vi "GetRaster_bu.vi"(0 "Galvo Array":refnum<class "Galvonometer.lvclass">[](array[class]), 1 "Scan.lvclass":refnum<class "Scan.lvclass">, 5 "error in (no error)":errorcluster) -> (15 "Galvo Array":dbl[][](array[numeric]), 19 "error IO":errorcluster)   [LabVIEW 2017]
uses:
  classes/Scans/Scan.lvclass
  classes/HardwareObjects/Galvonometer/Galvonometer.lvclass
  classes/Scans/Scan.lvclass/Scan.ctl
  classes/HardwareObjects/Galvonometer/Galvonometer.lvclass/Galvonometer.ctl
  classes/Scans/Read A scans.vi
  classes/Scans/Read B scans.vi
  classes/Scans/Read Bidirectional.vi
  classes/Scans/Read C scans.vi
  classes/Scans/Read Repeat B scans.vi
  classes/Scans/Read Scan Angle (degrees).vi
  classes/Scans/Read Scan Pattern.vi
  classes/Scans/Read X FOV (degrees).vi
  classes/Scans/Read X offset (degrees).vi
  classes/Scans/Read Y FOV (degrees).vi
  classes/Scans/Read Y offset (degrees).vi
  <vilib>/Analysis/1siggen.llb/Ramp Pattern by Samples.vi
  classes/HardwareObjects/Galvonometer/Read Output Scale Factor (V_degrees).vi
  <vilib>/Utility/file.llb/Write Delimited Spreadsheet (DBL).vi
  <vilib>/Analysis/NI_AALBase.lvlib
panel:
  in  "Read scan parameters":bool
  in  "Display Raster":bool
  out "Y offset (degrees)":dbl
  out "Y FOV (degrees)":dbl
  out "X offset (degrees)":dbl
  out "X FOV (degrees)":dbl
  out "Scan Pattern":string
  out "Scan Angle (degrees)":dbl
  out "Repeat B scans":dbl
  out "C scans":dbl
  out "Bidirectional":bool
  out "B scans":dbl
  out "A scans":dbl
  out "Raster":dbl[][](graph)
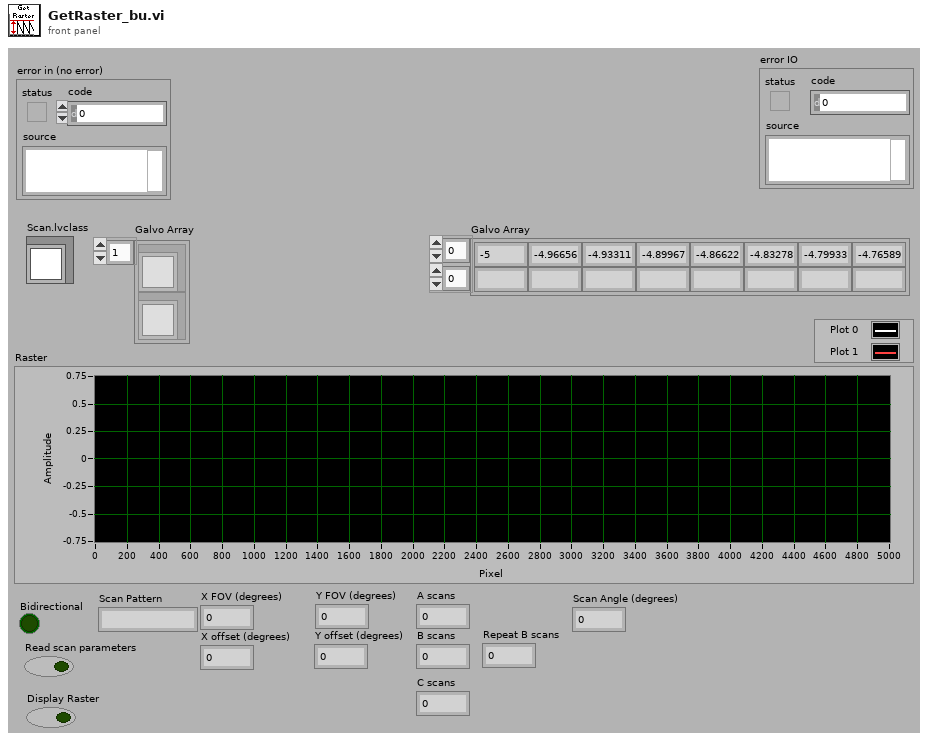
[diagram p1: front panel]
types:
  T1 = cluster{"X FOV (degrees)":dbl, "X offset (degrees)":dbl, "Y FOV (degrees)":dbl, "Y offset (degrees)":dbl}
  T2 = cluster{"X FOV (degrees)":dbl, "Y FOV (degrees)":dbl}
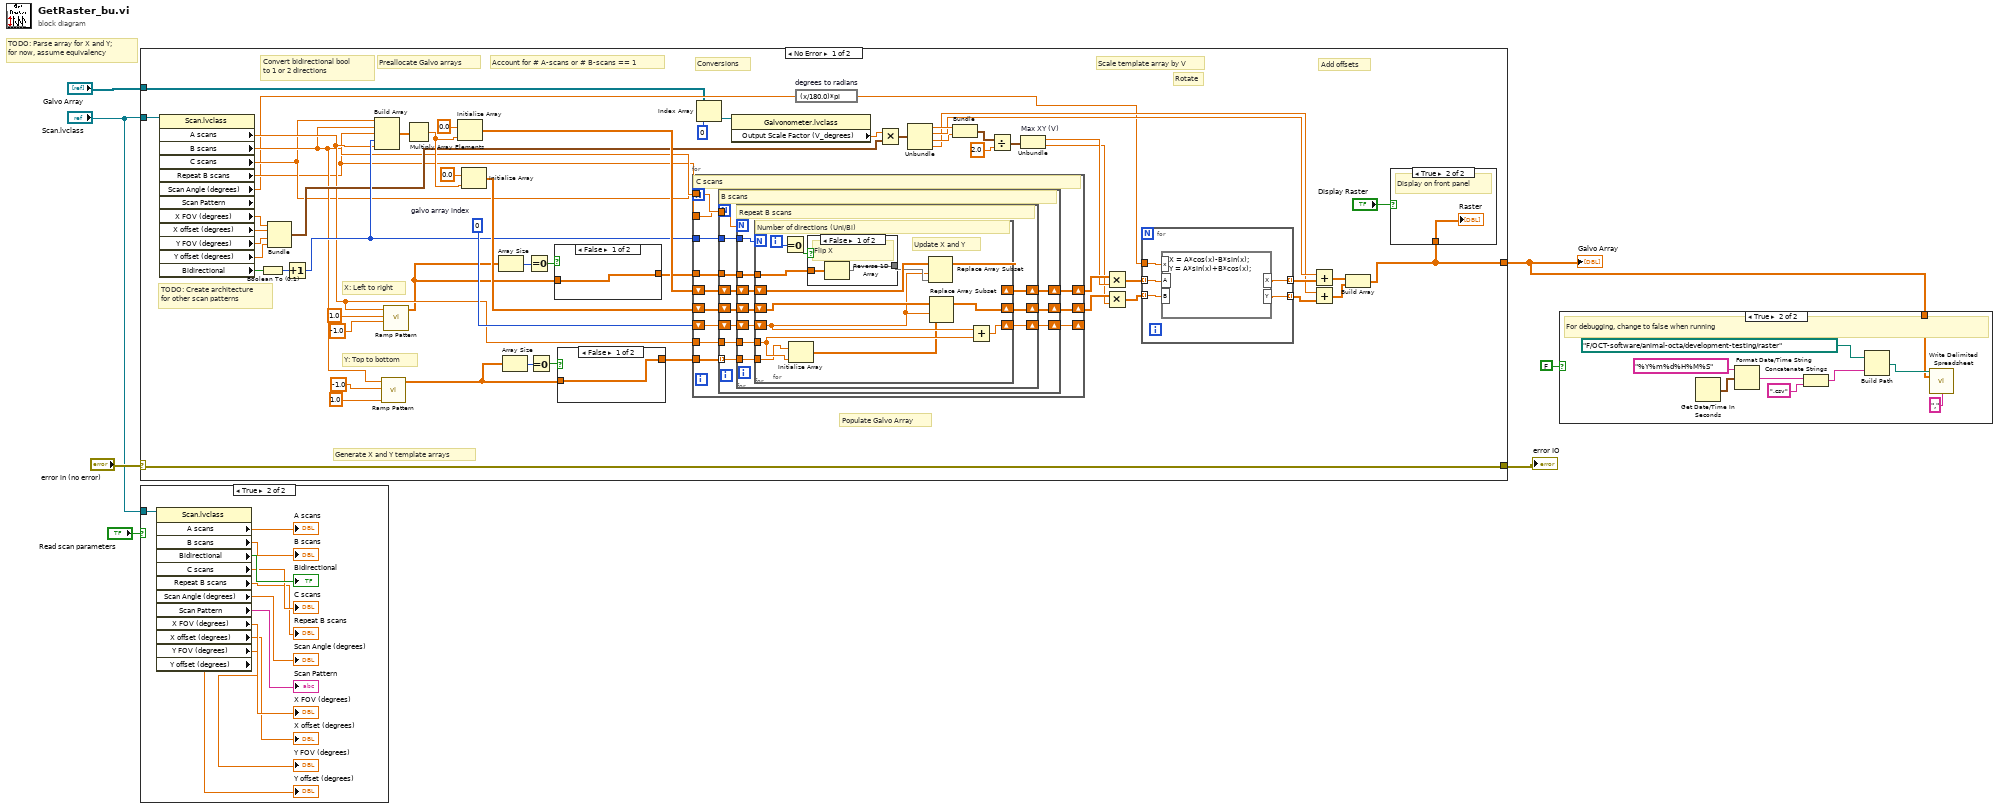
[diagram p0: block diagram]
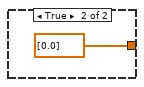
[diagram p3: hidden frame]
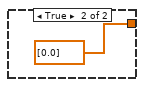
[diagram p4: hidden frame]
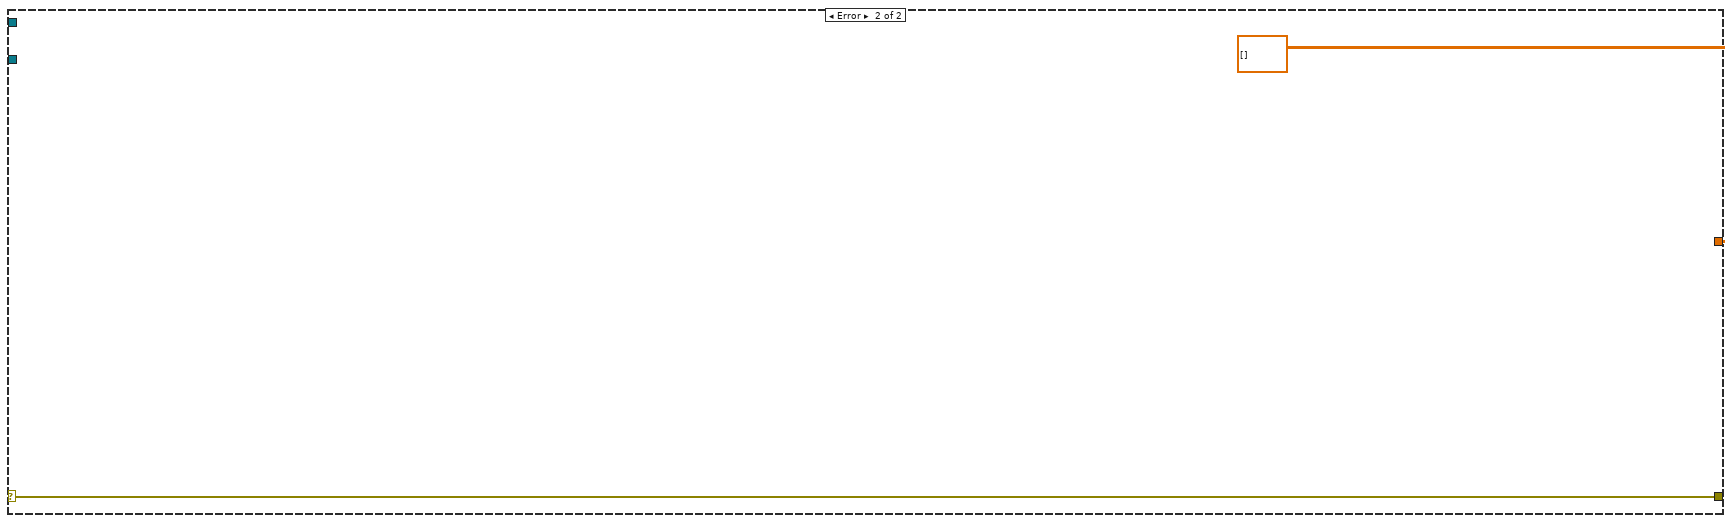
[diagram p7: hidden frame]
diagram:
  # "TODO: Parse array for X and Y;\nfor now, assume equivalency"
  n1 = case shown="No Error" "error in (no error)" {
    selector: "error in (no error)" -> [w66 w127]
    tunnel: [w66 w127] -> w7
    tunnel: [w9 dbl[][] []] -> w2
    tunnel: "Scan.lvclass" -> [w31 _]
    tunnel: "Galvo Array" -> [w22 _]
    frame No Error {
      w58 = 0  # galvo array index
      # "Account for # A-scans or # B-scans == 1"
      # "TODO: Create architecture\nfor other scan patterns"
      # "Convert bidirectional bool\nto 1 or 2 directions"
      # "Conversions"
      # "Add offsets"
      # "Rotate"
      # "Scale template array by V"
      # "Populate Galvo Array"
      # "Preallocate Galvo arrays"
      # "Y: Top to bottom"
      # "X: Left to right"
      # "Generate X and Y template arrays"
      n2 = property class="Scan.lvclass" props=["A scans", "B scans", "C scans", "Repeat B scans", "Scan Angle (degrees)", "Scan Pattern", "X FOV (degrees)", "X offset (degrees)", "Y FOV (degrees)", "Y offset (degrees)", "Bidirectional"](reference=w31) -> ("A scans"=w28:dbl, "B scans"=w27:dbl, "C scans"=w26:dbl, "Repeat B scans"=w25:dbl, "Scan Angle (degrees)"=w24:dbl, "X FOV (degrees)"=w32:dbl, "X offset (degrees)"=w33:dbl, "Y FOV (degrees)"=w34:dbl, "Y offset (degrees)"=w35:dbl, "Bidirectional"=w36:bool)  [unwired: 1 in, 3 out]
      n3 = Boolean To (0,1)(Boolean=w36) -> (0, 1=w37:i16)
      n4 = Bundle("X FOV (degrees)"=w32, "X offset (degrees)"=w33, "Y FOV (degrees)"=w34, "Y offset (degrees)"=w35) -> (w29:T1)  [unwired: 1 in]
      n5 = Increment(x=w37) -> (x+1=w30:i16)
      n6 = Build Array(w26, w27, w25, w30, w28) -> (w60:dbl[])
      n7 = call-poly <vilib>:"Ramp Pattern.vi"("start"=1.0, "end"=-1.0, "samples"=w27) -> ("Ramp Pattern"=w15:dbl[])  [unwired: 7 in, 1 out]
      n8 = call-poly <vilib>:"Ramp Pattern.vi"("start"=-1.0, "end"=1.0, "samples"=w28) -> ("Ramp Pattern"=w10:dbl[])  [unwired: 7 in, 1 out]
      n9 = Multiply Array Elements(1:w60) -> (0:w56:dbl)
      n10 = Initialize Array(0.0 ("element"), w56) -> (w59:dbl[])
      n11 = Initialize Array(0.0 ("element"), w56) -> (w55:dbl[])
      n12 = Array Size(array=w10) -> (size(s)=w12:i32)
      n13 = Array Size(array=w15) -> (size(s)=w16:i32)
      n14 = Equal To 0?(x=w12) -> (x = 0?=w11:bool)
      n15 = Equal To 0?(x=w16) -> (x = 0?=w17:bool)
      n16 = case shown="False" w11 {
        tunnel: w10 -> [w67 _]
        tunnel: [w67 dbl[] [0.0] ("Ramp Pattern")] -> w13
        frame False {
        }
        frame True {
        }
      }
      n17 = case shown="False" w17 {
        tunnel: w15 -> [w69 _]
        tunnel: [w69 dbl[] [0.0] ("Ramp Pattern")] -> w14
        frame False {
        }
        frame True {
        }
      }
      n18 = for {
        N: w26 -> [_]
        tunnel: w27 -> [w88]
        tunnel: w25 -> [w87]
        tunnel: w30 -> [w86]
        tunnel: w13 -> [w84]
        tunnel: w28 -> [w82]
        shift-right: [w78] -> _
        shift-left: w58 -> [w83]
        shift-right: [w81] -> w54
        shift-left: w59 -> [w85]
        shift-right: [w79] -> w53
        shift-left: w55 -> [w80]
        tunnel: w14 -> [w77]
        # "C scans"
        n19 = for {
          N: w88 -> [_]
          tunnel: w87 -> [w99]
          tunnel: w86 -> [w98]
          tunnel: w84 -> [w97]
          tunnel: w82 -> [w95]
          shift-right: [w91] -> w78
          shift-left: w83 -> [w96]
          shift-right: [w94] -> w81
          shift-left: w85 -> [w89]
          shift-right: [w92] -> w79
          shift-left: w80 -> [w93]
          tunnel: w77 -> [w90] mode=indexing
          # "B scans"
          n20 = for {
            N: w99 -> [_]
            tunnel: w98 -> [w109]
            tunnel: w97 -> [w108]
            tunnel: w95 -> [w106]
            shift-right: [w102] -> w91
            shift-left: w96 -> [w107]
            shift-right: [w105] -> w94
            shift-left: w89 -> [w100]
            shift-right: [w103] -> w92
            shift-left: w93 -> [w104]
            tunnel: w90 -> [w101]
            # "Repeat B scans"
            n21 = for {
              N: w109 -> [_]
              tunnel: w108 -> [w120]
              shift-right: [w115] -> w105
              shift-left: w100 -> [w119]
              tunnel: w106 -> [w117]
              shift-right: [w118] -> w102
              shift-left: w107 -> [w112]
              shift-right: [w113] -> w103
              shift-left: w104 -> [w114]
              tunnel: w101 -> [w111]
              i -> [w122]
              # "Update X and Y"
              # "Number of directions (Uni/Bi)"
              n22 = Equal To 0?(x=w122) -> (x = 0?=w121:bool)
              n23 = Initialize Array(w111, w117) -> (w110:dbl[])
              n24 = case shown="False" w121 {
                tunnel: w120 -> [w124 w125]
                tunnel: [w123 w125] -> w116
                frame False {
                  # "Flip X"
                  n25 = Reverse 1D Array(array=w124) -> (reversed array=w123:dbl[])
                }
                frame True {
                  # "Leave X as is"
                }
              }
              n26 = Replace Array Subset(array=w119, new element=w116, index=w112) -> (w115:dbl[])
              n27 = Replace Array Subset(array=w114, new element=w110, index=w112) -> (w113:dbl[])
              n28 = Add(x=w112, y=w117) -> (x+y=w118:dbl)
            }
          }
        }
      }
      n29 = Index Array(array=w22, index=0) -> (element=w23:refnum<class "Galvonometer.lvclass">)
      n30 = property class="Galvonometer.lvclass"(reference=w23) -> ("Output Scale Factor (V_degrees)"=w20:dbl)  [unwired: 1 in, 2 out]
      n31 = expression code="(x/180.0)*pi" "degrees to radians"(w24) -> (w8:dbl)
      n32 = Multiply(x=w20, y=w29) -> (x*y=w38:T1)
      n33 = Unbundle ("All in Volts")(w38) -> ("X FOV (degrees)"=w41:dbl, "X offset (degrees)"=w40:dbl, "Y FOV (degrees)"=w39:dbl, "Y offset (degrees)"=w18:dbl)
      n34 = Bundle("X FOV (degrees)"=w41, "Y FOV (degrees)"=w39) -> (w42:T2)  [unwired: 1 in]
      n35 = Divide(x=w42, y=2.0) -> (x/y=w44:T2)
      n36 = Unbundle "Max XY (V)"(w44) -> ("X FOV (degrees)"=w46:dbl, "Y FOV (degrees)"=w45:dbl)
      n37 = Multiply(x=w54, y=w46) -> (x*y=w52:dbl[])
      n38 = Multiply(x=w53, y=w45) -> (x*y=w51:dbl[])
      n39 = for {
        tunnel: w52 -> [w76] mode=indexing
        tunnel: w8 -> [w75]
        tunnel: [w74] -> w49 mode=indexing
        tunnel: w51 -> [w73] mode=indexing
        tunnel: [w72] -> w19 mode=indexing
        n40 = formula code="X = A*cos(x)-B*sin(x);\nY = A*sin(x)+B*cos(x);"("x"=w75, "A"=w76, "B"=w73) -> ("X"=w74:dbl, "Y"=w72:dbl)
      }
      n41 = Add(x=w40, y=w49) -> (x+y=w48:dbl[])
      n42 = Add(x=w18, y=w19) -> (x+y=w47:dbl[])
      n43 = Build Array(w48, w47) -> (w9:dbl[][])
      n44 = case shown="True" "Display Raster" {
        tunnel: w9 -> [_ w71]
        frame False {
        }
        frame True {
          # "Display on front panel"
          "Raster" <- w71
        }
      }
    }
    frame Error {
    }
  }
  "error IO" <- w7
  "Galvo Array" <- w2
  n45 = case shown="True" "Read scan parameters" {
    tunnel: "Scan.lvclass" -> [_ w139]
    frame False {
    }
    frame True {
      n46 = property class="Scan.lvclass"(reference=w139) -> ("A scans"=→"A scans":dbl, "B scans"=→"B scans":dbl, "Bidirectional"=→"Bidirectional":bool, "C scans"=→"C scans":dbl, "Repeat B scans"=→"Repeat B scans":dbl, "Scan Angle (degrees)"=→"Scan Angle (degrees)":dbl, "Scan Pattern"=→"Scan Pattern":string, "X FOV (degrees)"=→"X FOV (degrees)":dbl, "X offset (degrees)"=→"X offset (degrees)":dbl, "Y FOV (degrees)"=→"Y FOV (degrees)":dbl, "Y offset (degrees)"=→"Y offset (degrees)":dbl)  [unwired: 1 in, 2 out]
    }
  }
  n47 = case shown="True" FALSE {
    tunnel: w2 -> [_ w140]
    frame False {
    }
    frame True {
      # "For debugging, change to false when running"
      n48 = Get Date/Time In Seconds() -> (seconds since 1Jan1904=w148:timestamp)
      n49 = Format Date/Time String(time format string (%c)="%Y%m%d%H%M%S", seconds (now)=w148) -> (date/time string=w144:string)  [unwired: 1 in]
      n50 = Concatenate Strings(w144, ".csv" ("string")) -> (w143:string)
      n51 = Build Path(base path=path "F:/OCT-software/animal-octa/development-testing/raster", name or relative path=w143) -> (appended path=w141:path)
      n52 = call-poly <vilib>:"Write Delimited Spreadsheet.vi"("file path (dialog if empty)"=w141, "2D data"=w140, "delimiter (\\t)"="," ("delimiter (\\t)")) -> ()  [unwired: 11 in, 2 out]
    }
  }
